vi "Get SQL Formatted Value.vi"(8 "error in (no error)":errorcluster, 10 "Value":variant, 11 "Numeric Value in":refnum<class "Numeric Value.lvclass">) -> (0 "error out":errorcluster, 2 "SQL Formatted Value":string, 3 "Numeric Value out":refnum<class "Numeric Value.lvclass">)   [LabVIEW 2020, in "Composed Columns.lvlib" / "Numeric Value.lvclass"]
uses:
  Numeric Value.lvclass
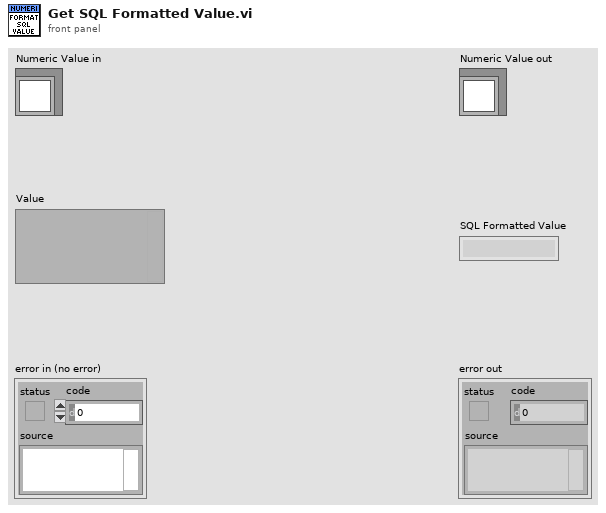
[diagram p1: front panel]
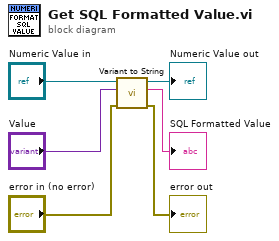
[diagram p0: block diagram]
diagram:
  n1 = call-dynamic "Variant to String.vi"("error in (no error)"="error in (no error)", "Variant"="Value", "Numeric Value in"="Numeric Value in") -> ("error out"=→"error out":errorcluster, "String"=→"SQL Formatted Value":string, "Numeric Value out"=→"Numeric Value out":refnum<class "Numeric Value.lvclass">)  [unwired: 6 in]
